vi "Send Message.vi"(8 "error in (no error)":errorcluster, 10 "Message":string, 11 "ProgressBar":refnum<class "ProgressBar.lvclass">) -> (0 "error out":errorcluster, 3 "ProgressBar out":refnum<class "ProgressBar.lvclass">)   [LabVIEW 2019, in "ProgressBar.lvclass"]
doc: "Send a message to be display on the splash screen (adding ... at the end gives it a good touch)"
uses:
  ProgressBar.lvclass
  ProgressBar.lvclass/ProgressBar.ctl
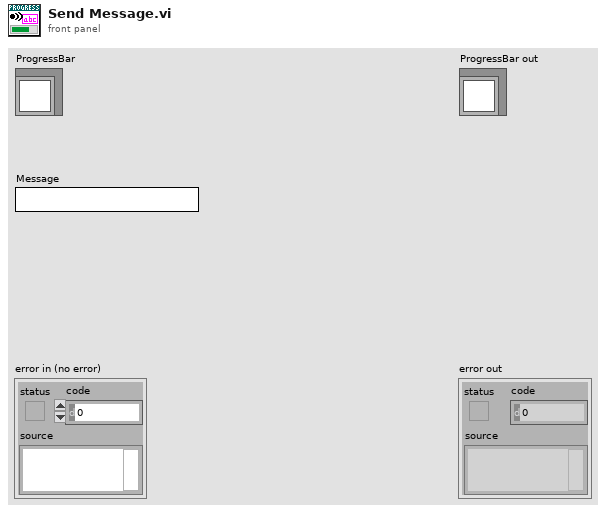
[diagram p1: front panel]
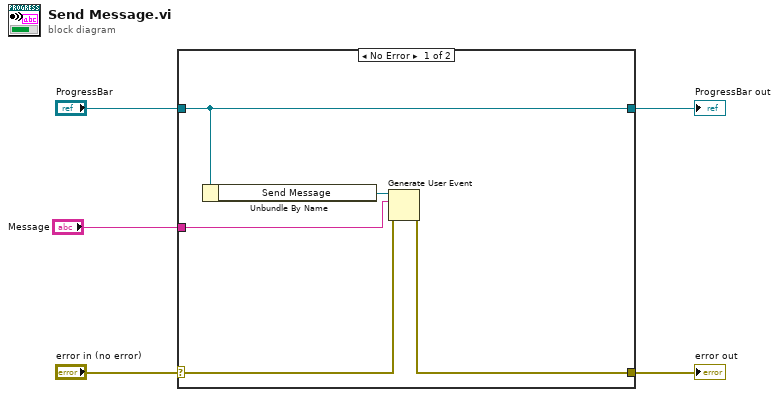
[diagram p0: block diagram]
diagram:
  n1 = case shown="No Error" "error in (no error)" {
    selector: "error in (no error)" -> [w8 w12]
    tunnel: [w7 w12] -> w4
    tunnel: [w6 w11] -> w2
    tunnel: "ProgressBar" -> [w6 w11]
    tunnel: "Message" -> [w9 _]
    frame No Error {
      n2 = Unbundle By Name(w6) -> ("Send Message"=w10:refnum<user-event>)
      n3 = Generate User Event(user event=w10, event data cluster=w9, error in=w8) -> (error out=w7:errorcluster)  [unwired: 1 in, 1 out]
    }
    frame Error {
    }
  }
  "error out" <- w4
  "ProgressBar out" <- w2
